vi "TareaValidacion.vi"() -> ()   [LabVIEW 2018]
panel:
  out "Mayor o Igual":string
  out "Numero Par":bool
  in  "Saber si un numero es Par":dbl=4.0
  out "Mayor Igual a Una Hora":bool
  out "Tiempo Segundos":dbl
  out "Tiempo Minutos":dbl
  out "Tiempo Horas":dbl
  in  "Tiempo Segundos":dbl=7000.0
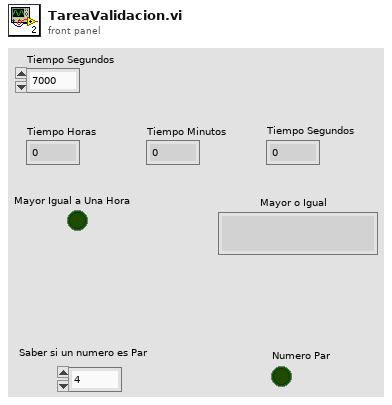
[diagram p1: front panel]
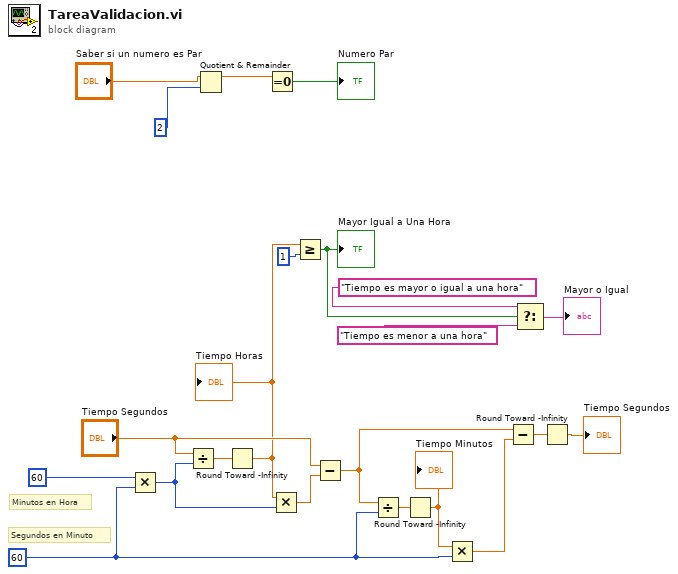
[diagram p0: block diagram]
diagram:
  w7 = 60
  # "Segundos en Minuto"
  # "Minutos en Hora"
  n1 = Multiply(x=60, y=w7) -> (x*y=w8:i32)
  n2 = Divide(x="Tiempo Segundos", y=w8) -> (x/y=w21:dbl)
  n3 = Quotient & Remainder(x="Saber si un numero es Par", y=2) -> (x-y*floor(x/y)=w3:dbl)  [unwired: 1 out]
  n4 = Round Toward -Infinity(1:w21) -> (0:w13:dbl)
  "Tiempo Horas" <- w13
  n5 = Equal To 0?(x=w3) -> (x = 0?=→"Numero Par":bool)
  n6 = Multiply(x=w13, y=w8) -> (x*y=w19:dbl)
  n7 = Greater Or Equal?(x=w13, y=1) -> (x >= y?=w11:bool)
  "Mayor Igual a Una Hora" <- w11
  n8 = Subtract(x="Tiempo Segundos", y=w19) -> (x-y=w16:dbl)
  n9 = Divide(x=w16, y=w7) -> (x/y=w18:dbl)
  n10 = Round Toward -Infinity(1:w18) -> (0:w17:dbl)
  "Tiempo Minutos" <- w17
  n11 = Multiply(x=w17, y=w7) -> (x*y=w5:dbl)
  n12 = Subtract(x=w16, y=w5) -> (x-y=w15:dbl)
  n13 = Select(t="Tiempo es mayor o igual a una hora", s=w11, f="Tiempo es menor a una hora") -> (s? t:f=→"Mayor o Igual":string)
  n14 = Round Toward -Infinity(1:w15) -> (0:→"Tiempo Segundos":dbl)
